vi "제목없음 1.vi"() -> ()   [LabVIEW 2014]
uses:
  <vilib>/myRIO/Instrument Drivers/Onboard IO/AI/vis/Read.vi
  <vilib>/myRIO/Instrument Drivers/Onboard IO/AI/vis/Smart Open.vi
  <vilib>/Utility/error.llb/Error Cluster From Error Code.vi
  <vilib>/myRIO/Common/Instrument Driver Framework/myRIO v1.0/AI/vis/myRIO v1.0 Read AI.vi
panel:
  out "Col01 (B/AI1 (Pin 5))":dbl
  out "Col02 (B/AI2 (Pin 7))":dbl
  in  "정지":bool
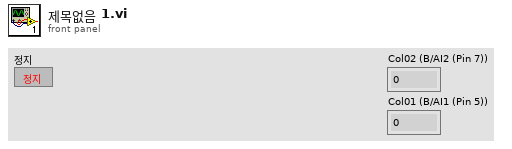
[diagram p1: front panel]
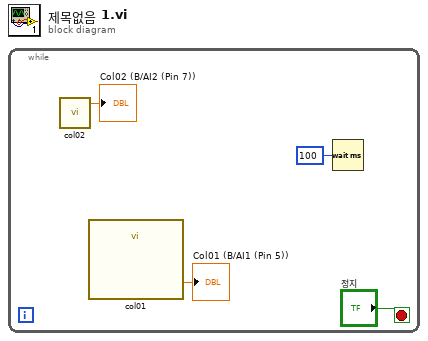
[diagram p0: block diagram]
diagram:
  n1 = while {
    stop <- "정지" stop-if-true
    n2 = call "col02.vi"() -> ("Col02 (B/AI2 (Pin 7))"=→"Col02 (B/AI2 (Pin 7))":dbl)  [unwired: 26 in, 1 out]
    n3 = call "col01.vi"() -> ("Col01 (B/AI1 (Pin 5))"=→"Col01 (B/AI1 (Pin 5))":dbl)  [unwired: 26 in, 1 out]
    n4 = Wait (ms)(milliseconds to wait=u32 100 ("대기 시간(ms)")) -> ()  [unwired: 1 out]
  }
